vi "Static ON OFF.vi"(8 "error in":errorcluster, 10 "ON":bool, 11 "TEC 1090 in":refnum<class "Meerstetter TEC.lvclass">) -> (0 "error out":errorcluster, 3 "TEC 1090 out":refnum<class "Meerstetter TEC.lvclass">)   [LabVIEW 2014, in "Meerstetter Lib.lvlib" / "Meerstetter TEC.lvclass"]
uses:
  Meerstetter TEC.lvclass
  Controls/Output Selection.ctl
  Configurable Device/Configurable Device.lvclass/Configurable Device.ctl
  Configurable Device/Write Device Active_.vi
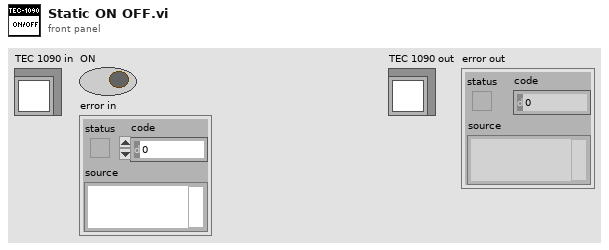
[diagram p1: front panel]
types:
  T1 = typedef "Meerstetter Lib.lvlib/Meerstetter TEC.lvclass/Output Selection.ctl" = enum16{"Static OFF", "Static ON", "Live OFF/ON", "HW Enable"}
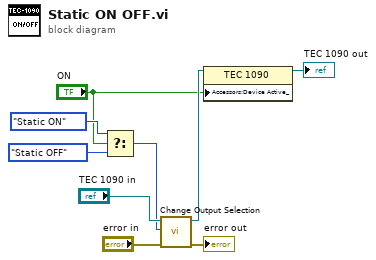
[diagram p0: block diagram]
diagram:
  n1 = Select(t=Output_Selection."Static ON", s="ON", f=Output_Selection."Static OFF" ("Output Selection")) -> (s? t:f=w7:T1)
  n2 = call "Change Output Selection.vi"("error in"="error in", "Output Selection"=w7, "TEC 1090 in"="TEC 1090 in") -> ("error out"=→"error out":errorcluster, "TEC 1090 out"=w3:refnum<class "Meerstetter TEC.lvclass">)  [unwired: 7 in]
  n3 = property class="TEC 1090"(reference=w3, "Accessors:Device Active_"="ON") -> (reference out=→"TEC 1090 out":refnum<class "Meerstetter TEC.lvclass">)  [unwired: 1 in, 1 out]
